vi "Increment Loop.vi"() -> ()   [LabVIEW 2016]
panel:
  out "x":dbl
  out "x+y":dbl
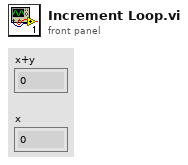
[diagram p1: front panel]
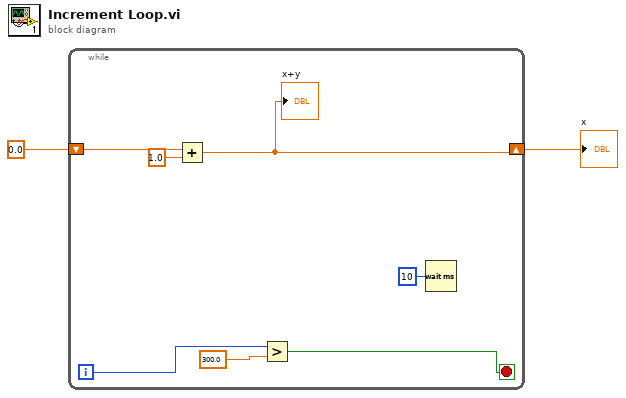
[diagram p0: block diagram]
diagram:
  n1 = while {
    shift-right: [w7] -> w1
    shift-left: 0.0 ("Numeric") -> [w9]
    i -> [w4]
    stop <- w3 stop-if-true
    n2 = Add(x=w9, y=1.0) -> (x+y=w7:dbl)
    "x+y" <- w7
    n3 = Greater?(x=w4, y=300.0) -> (0:w3:bool)
    n4 = Wait (ms)(milliseconds to wait=u32 10) -> ()  [unwired: 1 out]
  }
  "x" <- w1
